vi "configure.vi"(8 "error in (no error)":errorcluster, 11 "ILCSim1 in":refnum<class "ILCSim1.lvclass">) -> (0 "error out":errorcluster, 3 "ILCSim1 out":refnum<class "ILCSim1.lvclass">)   [LabVIEW 2013, in "ILCSim1.lvclass"]
uses:
  ILCSim1.lvclass
  <userlib>/Common/ILC/Configuration/ILC ADC.ctl
  <userlib>/Common/ILC/Configuration/InputChannels.ctl
  <userlib>/Common/ILC/Configuration/ScanRate_Hz_MultichannelOptions.ctl
  ILCSim1.lvclass/ILCSim1.ctl
  ConfigurationThisComponent/ConfigurationThisComponent.lvclass
  <userlib>/Common/ILC/Configuration/ILCConfiguration.lvlib
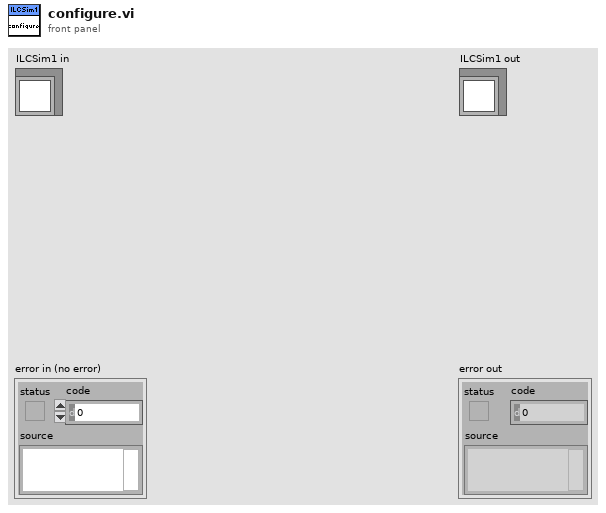
[diagram p1: front panel]
types:
  T1 = typedef "ILCCommon.lvlib/ILCConfiguration.lvlib/ILC ADC.ctl" = cluster{"Input Channels":T2, "Scan Rate (Hz) ":T3, "PGA Gain Coefficient":u8, "Reference Voltage Vref":dbl[unit], "Nominal Input Range in Counts":u32, "Preamplifier Gain":u8}
  T2 = typedef "ILCCommon.lvlib/ILCConfiguration.lvlib/InputChannels.ctl" = enum16{"Channel 0", "3 Channels", "5 Channels"}
  T3 = typedef "ILCCommon.lvlib/ILCConfiguration.lvlib/ScanRate_Hz_MultichannelOptions.ctl" = enum16{"50", "60", "100", "120", "200", "240", "300", "400", "480", "600", "1200", "2400", "4800"}
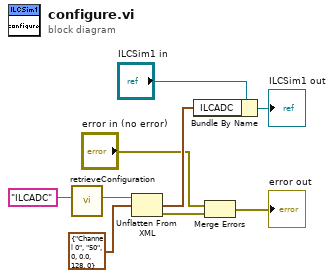
[diagram p0: block diagram]
diagram:
  n1 = call "retrieveConfiguration.vi"("configName"="ILCADC") -> ("xmlConfig"=w8:string)  [unwired: 8 in, 2 out]
  n2 = Unflatten From XML(xml string=w8, type=T1 {"Input Channels"=enum."Channel 0", "Scan Rate (Hz) "=enum."50", "PGA Gain Coefficient"=0, "Reference Voltage Vref"=0.0, "Nominal Input Range in Counts"=128, "Preamplifier Gain"=0} ("ILCADC")) -> (value=w6:T1, error out=w3:errorcluster)  [unwired: 1 in]
  n3 = Bundle By Name(cluster="ILCSim1 in", "ILCADC"=w6) -> (→"ILCSim1 out":refnum<class "ILCSim1.lvclass">)
  n4 = Merge Errors("error in (no error)", w3) -> (→"error out":errorcluster)
